vi "Abort Impl.vi"(8 "error in (no error)":errorcluster, 11 "Ludl Stage in":refnum<class "Ludl Stage.lvclass">) -> (0 "error out":errorcluster, 3 "Ludl Stage out":refnum<class "Ludl Stage.lvclass">)   [LabVIEW 2023, in "Ludl Stage.lvlib" / "Ludl Stage.lvclass"]
uses:
  Ludl Stage.lvclass
  Ludl Stage.lvclass/Ludl Stage.ctl
  Stage Controller/Stage Controller.lvlib
panel:
  out "Response":string
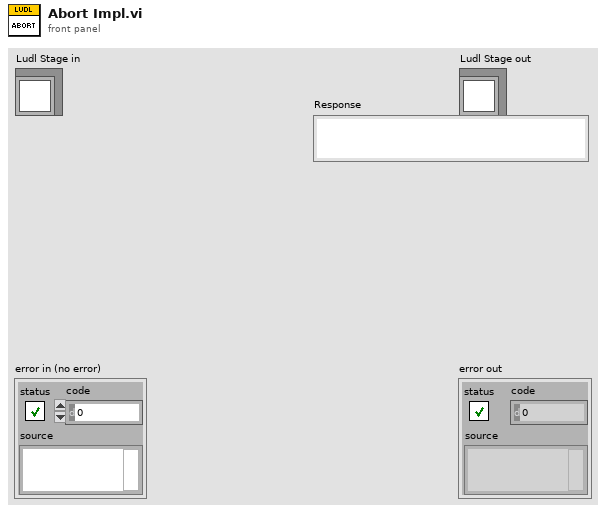
[diagram p1: front panel]
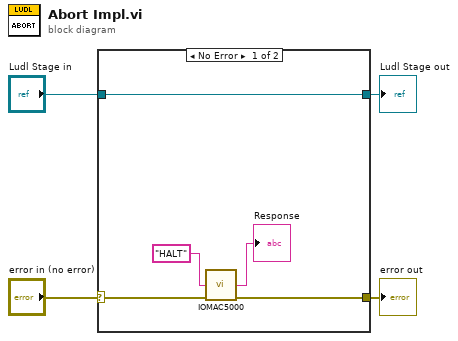
[diagram p0: block diagram]
diagram:
  n1 = case shown="No Error" "error in (no error)" {
    selector: "error in (no error)" -> [w7 w10]
    tunnel: [w8 w10] -> w4
    tunnel: "Ludl Stage in" -> [w6 w11]
    tunnel: [w6 w11] -> w1
    frame No Error {
      n2 = call "IOMAC5000.vi"("Command (to ctlr)"="HALT" ("true string"), "error in"=w7) -> ("Raw Response"=→"Response":string, "error out"=w8:errorcluster)  [unwired: 10 in, 2 out]
    }
    frame Error {
    }
  }
  "error out" <- w4
  "Ludl Stage out" <- w1
